vi "Ivium driver 1-02.vi"() -> ()   [LabVIEW 2020]
uses:
  <vilib>/Utility/file.llb/Write To Spreadsheet File (DBL).vi
  <vilib>/Utility/file.llb/Read From Spreadsheet File (DBL).vi
  Instance           3 25Saved   Ivium driver 1-02 .vi
  Instance           4 25Saved   Ivium driver 1-02 .vi
  Instance           2 25Saved   Ivium driver 1-02 .vi
  IVIUM_remdriver.lvlib
panel:
  out "Device serial number":string
  in  "Read device serial number":bool
  out "XY Graph":cluster{"Y":dbl[], "Y":dbl[]}[](graph)
  in  "Tab Control direct mode/method mode":enum32{"Direct Control", "Method control"}(tab)
  out "cell on":bool
  in  "Set Mux channel":i32
  in  "Tab Control Ac/external/bistat":enum32{"AC", "Extern", "BiStat"}(tab)
  in  "Amplitude":dbl caption="V" format="%_4f"
  in  "Frequency":dbl caption="Hz" format="%#_8f"
  out "Dig in 2":bool
  out "Dig in 1":bool
  in  "Dig out 1":bool
  in  "Read analog inputs":bool
  out "value /V":dbl[](array[numeric]) format="%_6g"
  in  "ch2":dbl caption="V" format="%_4g"
  in  "ch1":dbl caption="V" format="%_4p"
  in  "Read digital inputs":bool
  in  "Dig out 2":bool
  in  "Dig out 3":bool
  in  "Set Bi-Stat mode":enum16{"Standard", "Scanning"}(ring)
  in  "Get current":bool
  out "current 2":dbl caption="A" format="%_4g"
  in  "current range":T1(ring)=enum."1 mA"
  in  "offset potential":dbl caption="V" format="%_4g"
  in  "Get current":bool
  out "current":dbl caption="A" format="%_4g"
  in  "cell current":dbl caption="A" format="%_4p"
  in  "cell potential":dbl caption="V" format="%_3p"
  in  "Apply":enum16{"off", "on"}(ring)
  in  "Current range":T2(ring)=enum."10 mA"
  in  "Configuration":T3(ring)
  out "Device Status indicator":string
  in  "Get device status":bool
  out "cell-off button pressed":bool
  out "E_overload":bool
  out "Aninput1_overload":bool
  out "I_overload":bool
  in  "Get cell status":bool
  in  "Reset 2":bool
  out "potential":dbl caption="V" format="%_4g"
  in  "Get potential":bool
  in  "Set Filter":T4(ring)=enum."10 kHz"
  in  "Set Stability":T5(ring)=enum."Standard"
  in  "Reset 3":bool
  in  "Start/stop writing\ndata to spreadsheet file":bool
  in  "Start Chart":bool
  in  "Y Scale.Range:Minimum":dbl
  in  "Y Scale.Range:Maximum":dbl
  in  "stop":bool
  in  "Disconnect    Connect":bool
  # "I overload"
  # "Cell-off button pressed"
  # "E overload"
  # "Aninput1 overload"
  # "Ac signal"
  # "Analog input"
  # "Digital output"
  # "Analog output"
  # "ch1"
  # "ch2"
  # "ch3"
  # "ch4"
  # "ch5"
  # "Digital input"
  # "ch6"
  # "ch7"
  # "ch8"
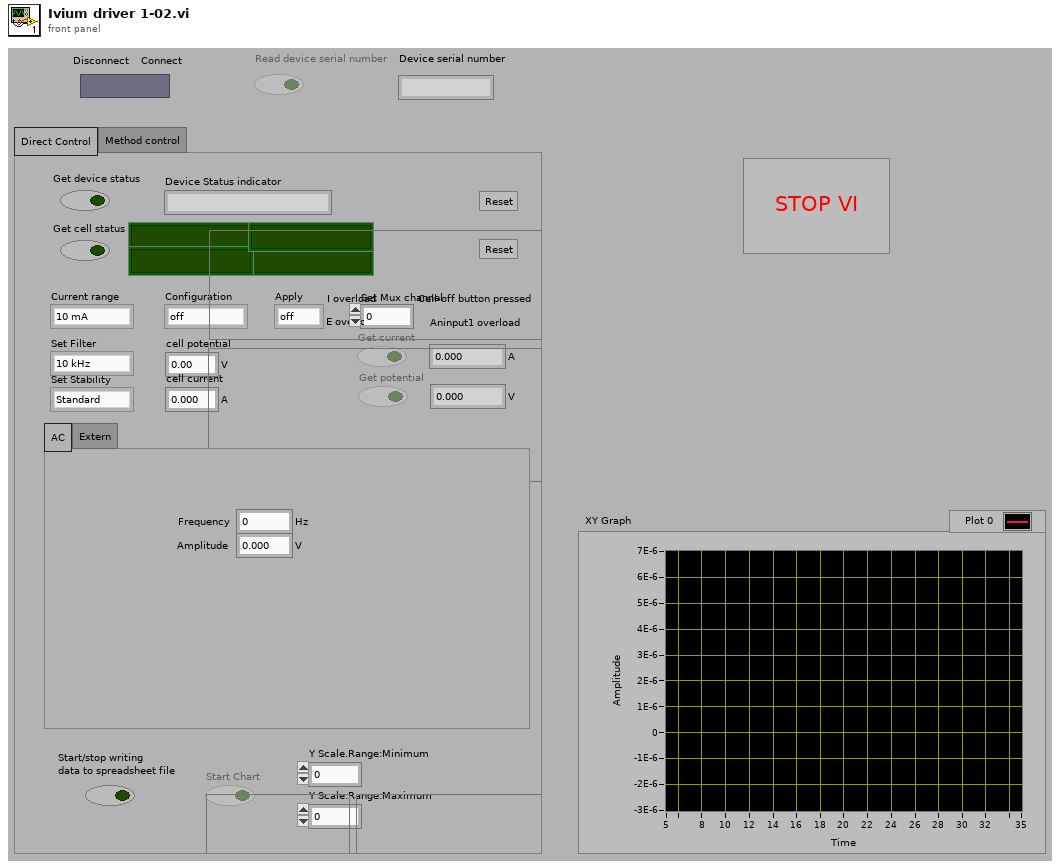
[diagram p1: front panel]
types:
  T1 = enum16{"10 mA", "1 mA", "100 uA", "10 uA", "1 uA", "100 nA", "10 nA", "1 nA", "100 pA", "10 pA", "1 pA"}
  T2 = enum16{"10 A", "1 A", "100 mA", "10 mA", "1 mA", "100 uA", "10 uA", "1 uA", "100 nA", "10 nA", "1 nA", "100 pA", "10 pA", "1 pA"}
  T3 = enum16{"off", "EStat4EL", "EStat2EL", "EStatDummy1", "EStatDummy2", "EStatDummy3", "EStatDummy4", "IStat4EL", "IStat2EL", "IStatDummy", "BiStat4EL", "BiStat2EL"}
  T4 = enum16{"1 MHz", "100 kHz", "10 kHz", "1 kHz", "10 Hz"}
  T5 = enum16{"High Speed", "Standard", "High Stability"}
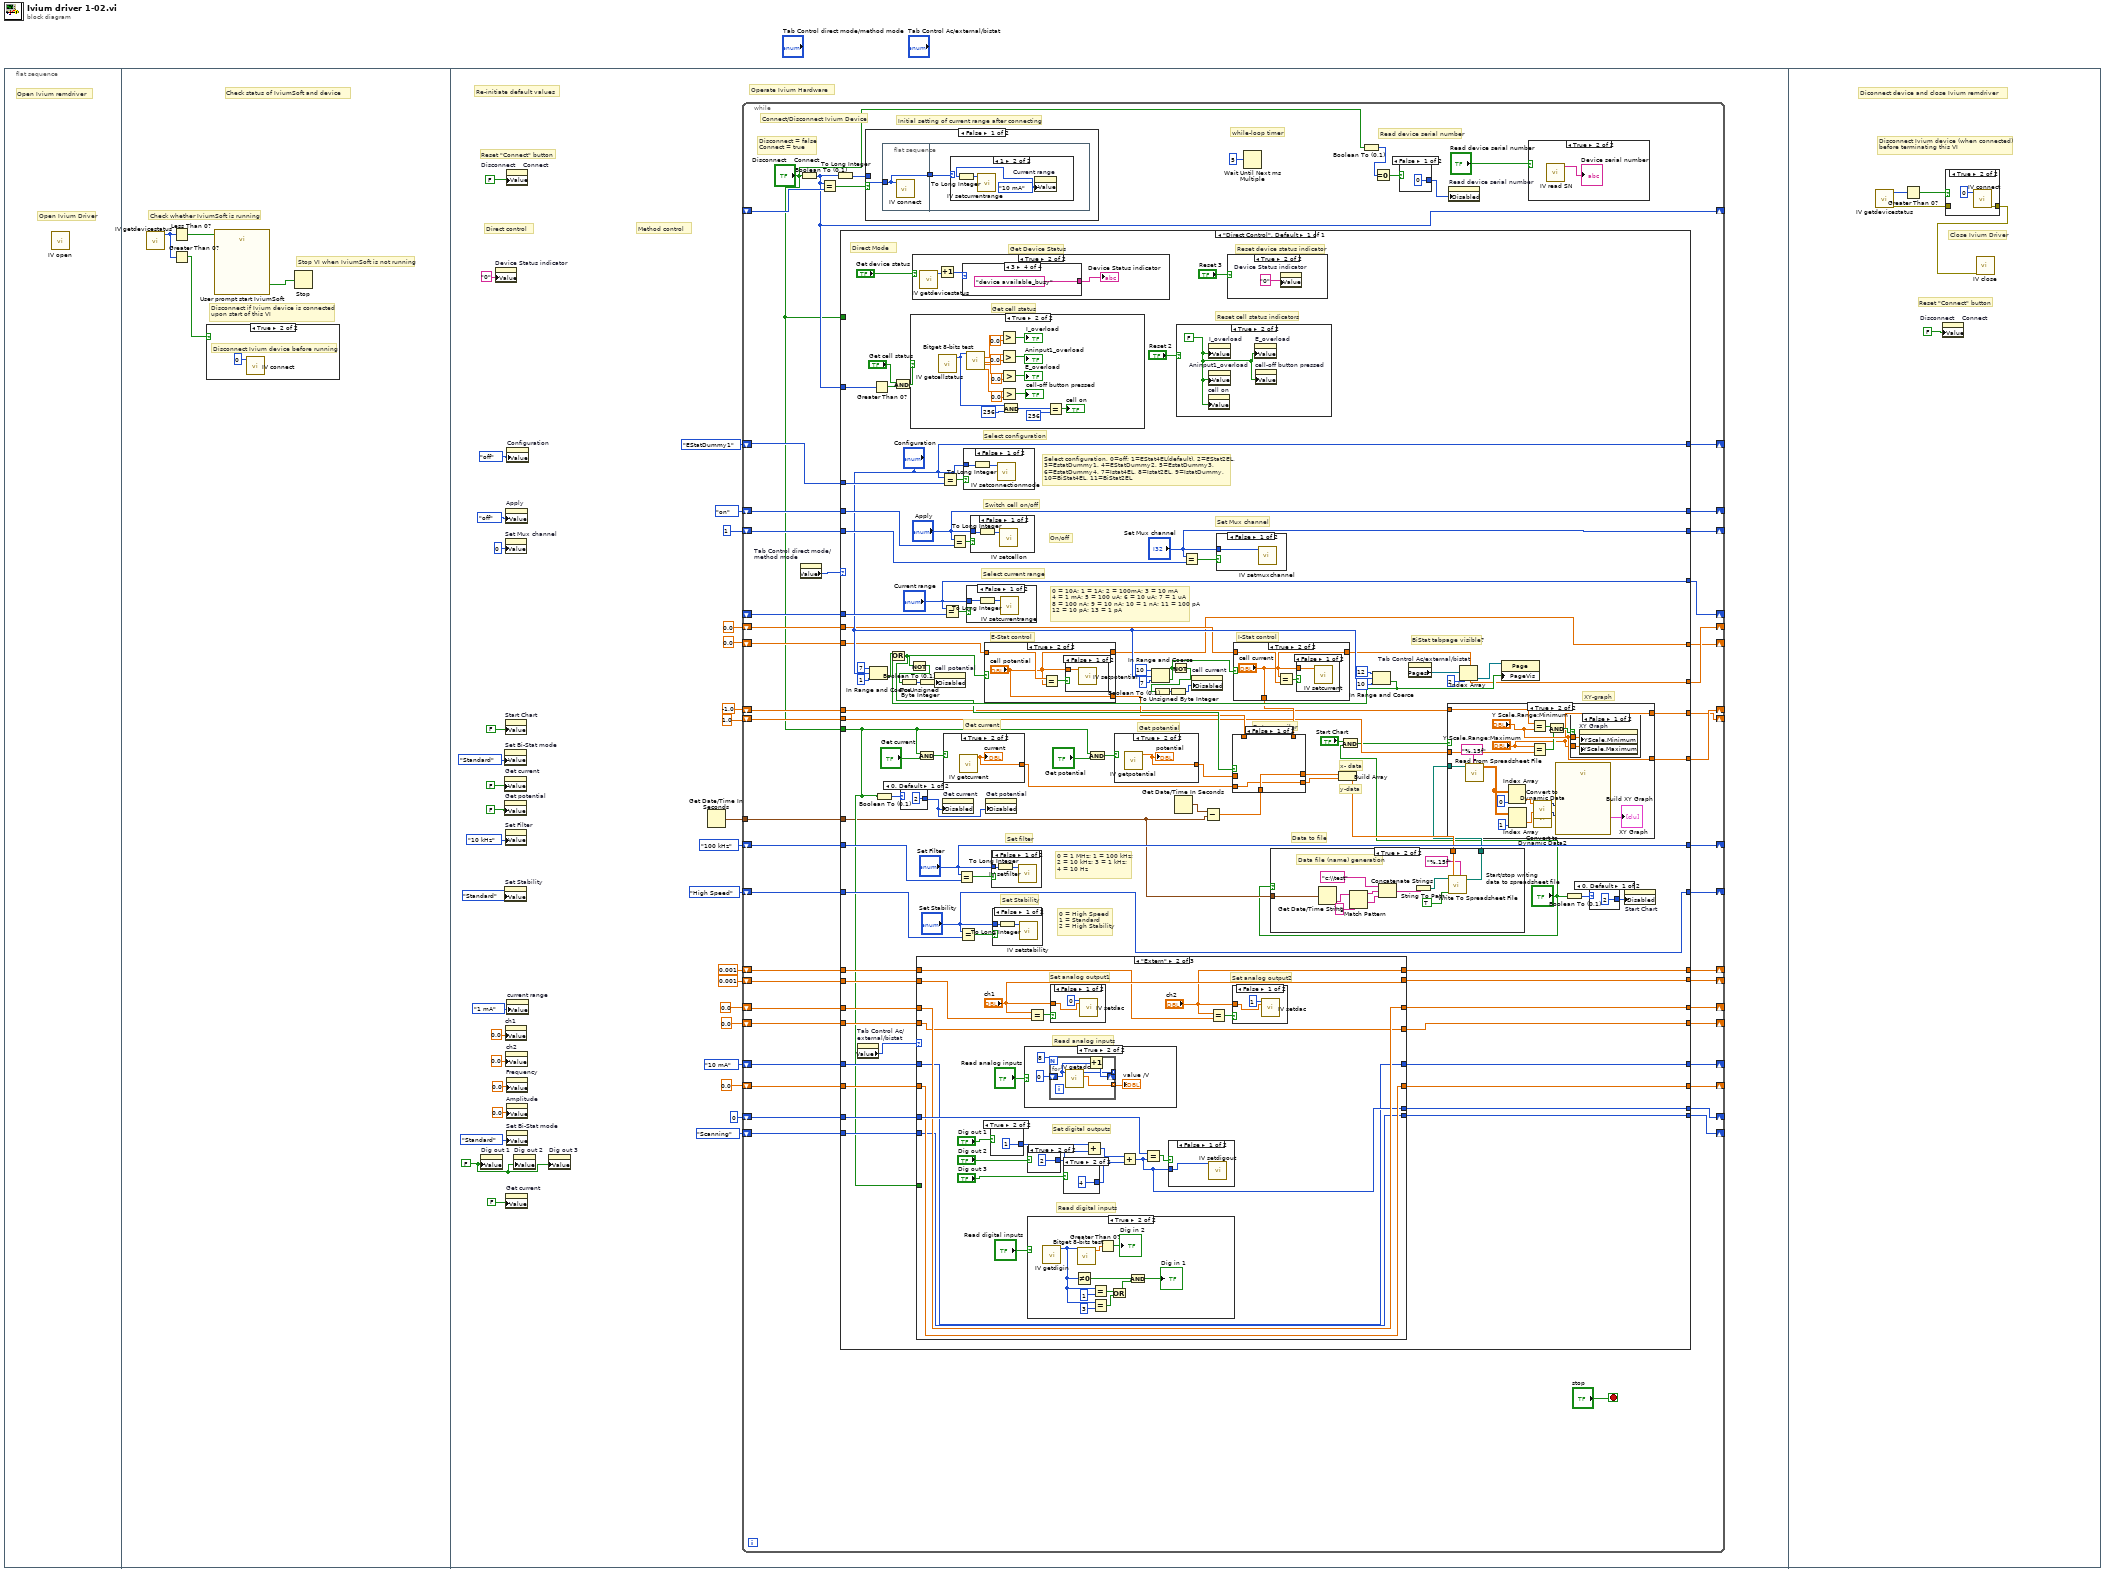
[diagram p0: block diagram]
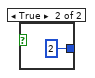
[diagram p4: hidden frame]
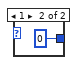
[diagram p5: hidden frame]
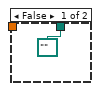
[diagram p6: hidden frame]
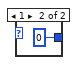
[diagram p10: hidden frame]
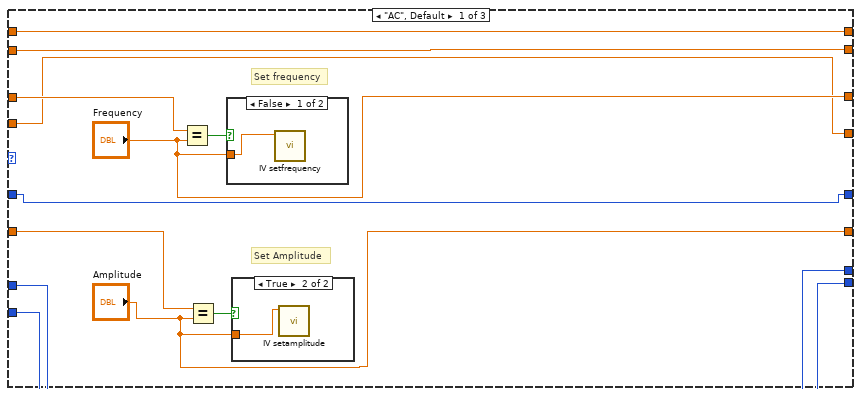
[diagram p12: hidden frame]
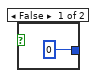
[diagram p16: hidden frame]
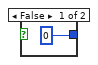
[diagram p17: hidden frame]
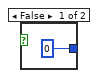
[diagram p18: hidden frame]
diagram:
  n1 = flat-sequence {
    frame #0 {
      # "Open Ivium remdriver"
      # "Open Ivium Driver"
      n2 = call "IV open.vi"() -> ()  [unwired: 10 in, 2 out]
    }
    frame #1 {
      # "Check status of IviumSoft and device"
      # "Stop VI when IviumSoft is not running"
      # "Disconnect if Ivium device is connected \nupon start of this VI"
      # "Check whether IviumSoft is running"
      n3 = call "IV getdevicestatus.vi"() -> ("return type"=w4:i32)  [unwired: 10 in, 1 out]
      n4 = Less Than 0?(x=w4) -> (x < 0?=w1:bool)
      n5 = Greater Than 0?(x=w4) -> (x > 0?=w3:bool)
      n6 = case shown="True" w3 {
        frame False {
        }
        frame True {
          # "Disconnect Ivium device before running"
          n7 = call "IV connect.vi"("devconnect"=0) -> ()  [unwired: 8 in, 3 out]
        }
      }
      n8 = call "User prompt start IviumSoft.vi"("Enable"=w1) -> ("OK"=w2:bool)  [unwired: 17 in, 1 out]
      n9 = Stop(stop? (T)=w2) -> ()
    }
    frame #2 {
      w12 = FALSE
      # "Method control"
      # "Direct control"
      # "Reset \"Connect\" button"
      # "Re-initiate default values"
      # "Operate Ivium Hardware"
      n10 = property on="Dig out 1" class="Bool (strict)"("Value"=w12) -> ()  [unwired: 2 in, 2 out]
      n11 = property on="Device Status indicator" class="Str"("Value"="0" ("Device Status indicator 2")) -> ()  [unwired: 2 in, 2 out]
      n12 = property on="Set Bi-Stat mode" class="Enum (strict)"("Value"=enum16{"Standard", "Scanning"}."Standard" ("Set Bi-Stat mode")) -> ()  [unwired: 2 in, 2 out]
      n13 = property on="Get current" class="Bool (strict)"("Value"=FALSE ("Get current")) -> ()  [unwired: 2 in, 2 out]
      n14 = property on="Get potential" class="Bool (strict)"("Value"=FALSE ("Get potential")) -> ()  [unwired: 2 in, 2 out]
      n15 = property on="Set Stability" class="Enum (strict)"("Value"=T5."Standard" ("Set Stability")) -> ()  [unwired: 2 in, 2 out]
      n16 = property on="Set Mux channel" class="DigNum (strict)"("Value"=0 ("Set Mux channel")) -> ()  [unwired: 2 in, 2 out]
      n17 = property on="Start Chart" class="Bool (strict)"("Value"=FALSE ("Start Chart")) -> ()  [unwired: 2 in, 2 out]
      n18 = property on="Set Filter" class="Enum (strict)"("Value"=T4."10 kHz" ("Set Filter")) -> ()  [unwired: 2 in, 2 out]
      n19 = property on="ch1" class="DigNum (strict)"("Value"=0.0 ("ch1")) -> ()  [unwired: 2 in, 2 out]
      n20 = property on="Apply" class="Enum (strict)"("Value"=enum16{"off", "on"}."off" ("Cell on/off")) -> ()  [unwired: 2 in, 2 out]
      n21 = property on="ch2" class="DigNum (strict)"("Value"=0.0 ("ch2")) -> ()  [unwired: 2 in, 2 out]
      n22 = property on="Get current" class="Bool (strict)"("Value"=FALSE ("Get current")) -> ()  [unwired: 2 in, 2 out]
      n23 = property on="Disconnect    Connect" class="Bool (strict)"("Value"=FALSE) -> ()  [unwired: 2 in, 2 out]
      n24 = property on="Frequency" class="DigNum (strict)"("Value"=0.0 ("Frequency")) -> ()  [unwired: 2 in, 2 out]
      n25 = property on="Amplitude" class="DigNum (strict)"("Value"=0.0 ("Amplitude")) -> ()  [unwired: 2 in, 2 out]
      n26 = property on="Set Bi-Stat mode" class="Enum (strict)"("Value"=enum16{"Standard", "Scanning"}."Standard" ("Set Bi-Stat mode")) -> ()  [unwired: 2 in, 2 out]
      n27 = property on="Configuration" class="Enum (strict)"("Value"=T3."off" ("Configuration")) -> ()  [unwired: 2 in, 2 out]
      n28 = property on="current range" class="Enum (strict)"("Value"=T1."1 mA" ("current range")) -> ()  [unwired: 2 in, 2 out]
      n29 = property on="Dig out 2" class="Bool (strict)"("Value"=w12) -> ()  [unwired: 2 in, 2 out]
      n30 = property on="Dig out 3" class="Bool (strict)"("Value"=w12) -> ()  [unwired: 2 in, 2 out]
      n31 = Get Date/Time In Seconds() -> (seconds since 1Jan1904=w9:timestamp)
      n32 = while {
        shift-right: [w61] -> _
        shift-left: _ -> [w91]
        shift-right: [w84] -> _
        shift-left: _ -> [w89]
        shift-right: [w87] -> _
        shift-left: T3."EStatDummy1" ("Configuration") -> [w88]
        shift-right: [w86] -> _
        shift-left: enum16{"off", "on"}."on" ("Apply") -> [w85]
        shift-right: [w82] -> _
        shift-left: T1."10 mA" ("current range") -> [w81]
        shift-right: [w79] -> _
        shift-left: T4."100 kHz" ("Set Filter") -> [w80]
        shift-right: [w77] -> _
        shift-left: T5."High Speed" ("Set Stability") -> [w78]
        shift-right: [w76] -> _
        shift-left: enum16{"Standard", "Scanning"}."Scanning" ("Set Bi-Stat mode") -> [w75]
        shift-right: [w73] -> _
        shift-left: 0.001 ("ch1") -> [w74]
        shift-right: [w72] -> _
        shift-left: 0.001 ("ch2") -> [w71]
        shift-right: [w70] -> _
        shift-left: 1 ("Set Mux channel") -> [w69]
        shift-right: [w60] -> _
        shift-left: 0 -> [w67]
        shift-right: [w65] -> _
        shift-left: 0.0 -> [w66]
        shift-right: [w63] -> _
        shift-left: 0.0 -> [w64]
        shift-right: [w58] -> _
        shift-left: 0.0 -> [w59]
        shift-right: [w56] -> _
        shift-left: 0.0 -> [w57]
        shift-right: [w54] -> _
        shift-left: 0.0 -> [w55]
        tunnel: w9 -> [w53]
        shift-right: [w50] -> _
        shift-left: -1.0 -> [w52]
        shift-right: [w49] -> _
        shift-left: 1.0 -> [w51]
        stop <- "stop" stop-if-true
        # "Read device serial number"
        # "while-loop timer"
        # "Initial setting of current range after connecting"
        # "Disconnect = false\nConnect = true"
        # "Connect/Disconnect Ivium Device"
        n33 = Boolean To (0,1)(Boolean="Disconnect    Connect") -> (0, 1=w61:i16)
        n34 = property on="Tab Control direct mode/\nmethod mode" class="TabCtl (strict)"() -> ("Value"=w48:enum32{"Direct Control", "Method control"})  [unwired: 2 in, 2 out]
        n35 = Equal?(x=w61, y=w91) -> (x = y?=w90:bool)
        n36 = To Long Integer(number=w61) -> (32bit integer=w62:i32)
        n37 = case shown="\"Direct Control\", Default" w48 {
          tunnel: w89 -> [w185]
          tunnel: w88 -> [w183]
          tunnel: ["Configuration"] -> w87
          tunnel: ["Apply"] -> w86
          tunnel: w85 -> [w180]
          tunnel: "Disconnect    Connect" -> [w123]
          tunnel: ["Current range"] -> w84
          tunnel: w61 -> [w169]
          tunnel: [w133] -> w82
          tunnel: w81 -> [w134]
          tunnel: w80 -> [w159]
          tunnel: ["Set Filter"] -> w79
          tunnel: w78 -> [w157]
          tunnel: ["Set Stability"] -> w77
          tunnel: [w131] -> w76
          tunnel: w75 -> [w132]
          tunnel: w74 -> [w155]
          tunnel: [w154] -> w73
          tunnel: [w153] -> w72
          tunnel: w71 -> [w152]
          tunnel: ["Set Mux channel"] -> w70
          tunnel: w69 -> [w150]
          tunnel: w67 -> [w145]
          tunnel: w66 -> [w144]
          tunnel: [w143] -> w65
          tunnel: w64 -> [w142]
          tunnel: [w141] -> w63
          tunnel: [w130] -> w60
          tunnel: w59 -> [w129]
          tunnel: [w128] -> w58
          tunnel: w57 -> [w114]
          tunnel: [w113] -> w56
          tunnel: w55 -> [w112]
          tunnel: [w111] -> w54
          tunnel: w53 -> [w106]
          tunnel: w52 -> [w105]
          tunnel: w51 -> [w104]
          tunnel: [w103] -> w50
          tunnel: [w102] -> w49
          tunnel: "Disconnect    Connect" -> [_]
          frame "Direct Control", Default {
            # "XY-graph"
            # "Data to file"
            # "Data compiler"
            # "y-data"
            # "x- data"
            # "BiStat tabpage visible?"
            # "Get potential"
            # "Get current"
            # "Set Mux channel"
            # "Reset device status indicator"
            # "0 = High Speed\n1 = Standard \n2 = High Stability"
            # "Set Stability"
            # "0 = 1 MHz; 1 = 100 kHz; \n2 = 10 kHz; 3 = 1 kHz; \n4 = 10 Hz"
            # "Set filter"
            # "On/off"
            # "I-Stat control"
            # "E-Stat control"
            # "Reset cell status indicators"
            # "Get cell status"
            # "Get Device Status"
            # "0 = 10A; 1 = 1A; 2 = 100mA; 3 = 10 mA\n4 = 1 mA; 5 = 100 uA; 6 = 10 uA; 7 = 1 uA\n8 = 100 nA; 9 = 10 nA; 10 = 1 nA; 11 = 100 pA\n12 = 10 pA; 13 = 1 pA"
            # "Select configuration"
            # "Direct Mode"
            # "Switch cell on/off"
            # "Select current range"
            # "Select configuration, 0=off; 1=EStat4EL(default), 2=EStat2EL, 3=EstatDummy1, 4=EStatDummy2, 5=EstatDummy3, 6=EstatDummy4, 7=Istat4EL, 8=Istat2EL, 9=IstatDummy, 10=BiStat4EL, 11=BiStat2EL"
            n38 = property on="Tab Control Ac/\nexternal/bistat" class="TabCtl (strict)"() -> ("Value"=w127:enum32{"AC", "Extern", "BiStat"})  [unwired: 2 in, 2 out]
            n39 = In Range and Coerce(upper limit=u16 7, x="Configuration", lower limit=u16 1) -> (In Range?=w162:bool)  [unwired: 1 out]
            n40 = Greater Than 0?(x=w169) -> (x > 0?=w170:bool)
            n41 = Boolean To (0,1)(Boolean=w123) -> (0, 1=w147:i16)
            n42 = And(x="Get cell status", y=w170) -> (x .and. y?=w172:bool)
            n43 = case shown="0, Default" w147 {
              tunnel: [u8 2 u8 0] -> w146
              frame 0, Default {
              }
              frame 1 {
              }
            }
            n44 = case shown="True" w172 {
              frame False {
              }
              frame True {
                n45 = call "IV getcellstatus.vi"() -> ("devcellstatus out"=w336:i32)  [unwired: 9 in, 2 out]
                n46 = call "Bitget 8-bits test.vi"("x"=w336) -> ("c"=w341:dbl, "e"=w339:dbl, "f"=w340:dbl, "h"=w337:dbl)  [unwired: 19 in, 4 out]
                n47 = Greater?(x=w341, y=0.0) -> (0:→"I_overload":bool)
                n48 = Greater?(x=w339, y=0.0) -> (0:→"Aninput1_overload":bool)
                n49 = Greater?(x=w340, y=0.0) -> (0:→"E_overload":bool)
                n50 = Greater?(x=w337, y=0.0) -> (0:→"cell-off button pressed":bool)
                n51 = And(x=w336, y=256) -> (x .and. y?=w334:i32)
                n52 = Equal?(x=w334, y=256) -> (x = y?=→"cell on":bool)
              }
            }
            n53 = case shown="True" "Get device status" {
              frame False {
                (unwired) 0
              }
              frame True {
                n54 = call "IV getdevicestatus.vi"() -> ("return type"=w351:i32)  [unwired: 10 in, 1 out]
                n55 = Increment(x=w351) -> (x+1=w350:i32)
                n56 = case shown="3" w350 {
                  tunnel: ["no IviumSoft" "device not connected" "device available_idle" "device available_busy"] -> w349
                  frame 0, Default {
                  }
                  frame 1 {
                  }
                  frame 2 {
                  }
                  frame 3 {
                  }
                }
                "Device Status indicator" <- w349
              }
            }
            n57 = case shown="\"Extern\"" w127 {
              tunnel: w155 -> [w240 w265 w306]
              tunnel: [w240 "ch1" w306] -> w154
              tunnel: [w241 "ch2" w307] -> w153
              tunnel: w152 -> [w241 w261 w307]
              tunnel: w145 -> [w231 w250 w303]
              tunnel: w144 -> [w238 w248 w305]
              tunnel: ["Frequency" w248 w305] -> w143
              tunnel: w142 -> [w235 w249 w304]
              tunnel: ["Amplitude" w249 w304] -> w141
              tunnel: w134 -> [w233 w245 w311]
              tunnel: [w233 w245 "current range"] -> w133
              tunnel: w132 -> [w232 w247 w309]
              tunnel: [w232 w247 "Set Bi-Stat mode"] -> w131
              tunnel: [w231 w246 w303] -> w130
              tunnel: w129 -> [w230 w244 w299]
              tunnel: [w230 w244 "offset potential"] -> w128
              tunnel: w123 -> [_ _ w295]
              frame "AC", Default {
                # "Set Amplitude"
                # "Set frequency"
                n58 = Equal?(x=w238, y="Frequency") -> (x = y?=w239:bool)
                n59 = Equal?(x=w235, y="Amplitude") -> (x = y?=w236:bool)
                n60 = case shown="False" w239 {
                  tunnel: "Frequency" -> [w243 _]
                  frame False {
                    n61 = call "IV setfrequency.vi"("value"=w243) -> ()  [unwired: 8 in, 3 out]
                  }
                  frame True {
                  }
                }
                n62 = case shown="True" w236 {
                  tunnel: "Amplitude" -> [_ w242]
                  frame False {
                  }
                  frame True {
                    n63 = call "IV setamplitude.vi"("value"=w242) -> ()  [unwired: 8 in, 3 out]
                  }
                }
              }
              frame "Extern" {
                # "Read digital inputs"
                # "Set digital outputs"
                # "Read analog inputs"
                # "Set analog output2"
                # "Set analog output1"
                n64 = case shown="True" "Dig out 1" {
                  tunnel: [0 1] -> w255
                  frame False {
                  }
                  frame True {
                  }
                }
                n65 = case shown="True" "Read analog inputs" {
                  frame False {
                  }
                  frame True {
                    n66 = for {
                      N: 8 -> [_]
                      shift-right: [w290] -> _
                      shift-left: 0 -> [w289]
                      tunnel: [w288] -> w284 mode=indexing
                      tunnel: [w287] -> _ mode=indexing
                      n67 = call "IV getadc.vi"("channr"=w289) -> ("value out"=w288:dbl, "channr out"=w287:i32)  [unwired: 7 in, 2 out]
                      n68 = Increment(x=w289) -> (x+1=w290:i32)
                    }
                    "value /V" <- w284
                  }
                }
                n69 = case shown="True" "Dig out 2" {
                  tunnel: [0 2] -> w254
                  frame False {
                  }
                  frame True {
                  }
                }
                n70 = case shown="True" "Read digital inputs" {
                  frame False {
                  }
                  frame True {
                    n71 = call "IV getdigin.vi"() -> ("value out"=w281:i32)  [unwired: 9 in, 2 out]
                    n72 = Not Equal To 0?(x=w281) -> (x != 0?=w276:bool)
                    n73 = call "Bitget 8-bits test.vi"("x"=w281) -> ("b"=w274:dbl)  [unwired: 19 in, 7 out]
                    n74 = Equal?(x=w281, y=1) -> (x = y?=w279:bool)
                    n75 = Equal?(x=w281, y=3) -> (x = y?=w278:bool)
                    n76 = Greater Than 0?(x=w274) -> (x > 0?=→"Dig in 2":bool)
                    n77 = Or(x=w279, y=w278) -> (x .or. y?=w277:bool)
                    n78 = And(x=w276, y=w277) -> (x .and. y?=→"Dig in 1":bool)
                  }
                }
                n79 = Equal?(x="ch1", y=w265) -> (x = y?=w266:bool)
                n80 = case shown="False" w266 {
                  tunnel: "ch1" -> [w293 _]
                  frame False {
                    n81 = call "IV setdac.vi"("value"=w293, "channr"=0) -> ()  [unwired: 6 in, 4 out]
                  }
                  frame True {
                  }
                }
                n82 = case shown="True" "Dig out 3" {
                  tunnel: [0 4] -> w252
                  frame False {
                  }
                  frame True {
                  }
                }
                n83 = Add(x=w255, y=w254) -> (x+y=w253:i32)
                n84 = Add(x=w253, y=w252) -> (x+y=w246:i32)
                n85 = Equal?(x=w250, y=w246) -> (x = y?=w251:bool)
                n86 = case shown="False" w251 {
                  tunnel: w246 -> [w267 _]
                  frame False {
                    n87 = call "IV setdigout.vi"("value"=w267) -> ()  [unwired: 8 in, 3 out]
                  }
                  frame True {
                  }
                }
                n88 = Equal?(x="ch2", y=w261) -> (x = y?=w263:bool)
                n89 = case shown="False" w263 {
                  tunnel: "ch2" -> [w291 _]
                  frame False {
                    n90 = call "IV setdac.vi"("value"=w291, "channr"=1) -> ()  [unwired: 6 in, 4 out]
                  }
                  frame True {
                  }
                }
              }
              frame "BiStat" {
                # "Bi-Stat mode:\n0 = standard\n1 = scanning"
                # "Bi-Stat current ranges:\n0 = 10 mA; 1 = 1 mA;\n2 = 100 uA; 3 = 10 uA;\n4 = 1 uA; 5 = 100 nA;\n6 = 10 nA; 7 = 1 nA;\n8 = 100 pA; 9 = 10 pA;\n10 = 1 pA"
                # "Bi-Stat control"
                n91 = Equal?(x=w299, y="offset potential") -> (x = y?=w300:bool)
                n92 = Equal?(x="current range", y=w311) -> (x = y?=w302:bool)
                n93 = Equal?(x="Set Bi-Stat mode", y=w309) -> (x = y?=w301:bool)
                n94 = case shown="True" w300 {
                  tunnel: "offset potential" -> [_ w313]
                  frame False {
                  }
                  frame True {
                    n95 = call "IV setpotential WE2.vi"("value"=w313) -> ()  [unwired: 8 in, 3 out]
                  }
                }
                n96 = case shown="False" w302 {
                  tunnel: "current range" -> [w316 _]
                  frame False {
                    n97 = To Long Integer(number=w316) -> (32bit integer=w317:i32)
                    n98 = call "IV setcurrentrange WE2.vi"("value"=w317) -> ()  [unwired: 8 in, 3 out]
                  }
                  frame True {
                  }
                }
                n99 = case shown="True" w301 {
                  tunnel: "Set Bi-Stat mode" -> [_ w314]
                  frame False {
                  }
                  frame True {
                    n100 = To Long Integer(number=w314) -> (32bit integer=w315:i32)
                    n101 = call "IV setbistatmode.vi"("value"=w315) -> ()  [unwired: 8 in, 3 out]
                  }
                }
                n102 = And(x=w295, y="Get current") -> (x .and. y?=w296:bool)
                n103 = case shown="True" w296 {
                  frame False {
                  }
                  frame True {
                    n104 = call "IV getcurrent WE2.vi"() -> ("value out"=→"current 2":dbl)  [unwired: 9 in, 2 out]
                  }
                }
              }
            }
            n105 = And(x=w123, y="Get current") -> (x .and. y?=w179:bool)
            n106 = Equal?(x="Configuration", y=w183) -> (x = y?=w184:bool)
            n107 = property on="Get current" class="Bool (strict)"("Disabled"=w146) -> ()  [unwired: 2 in, 2 out]
            n108 = Equal?(x="Current range", y=w185) -> (x = y?=w186:bool)
            n109 = case shown="True" w179 {
              tunnel: [0.0 ("value out") w363] -> w118
              frame False {
              }
              frame True {
                n110 = call "IV getcurrent.vi"() -> ("value out"=w363:dbl)  [unwired: 9 in, 2 out]
                "current" <- w363
              }
            }
            n111 = Equal?(x="Apply", y=w180) -> (x = y?=w182:bool)
            n112 = Equal?(x="Set Filter", y=w159) -> (x = y?=w122:bool)
            n113 = Equal?(x="Set Stability", y=w157) -> (x = y?=w158:bool)
            n114 = case shown="False" w184 {
              tunnel: "Configuration" -> [w366 _]
              frame False {
                n115 = To Long Integer(number=w366) -> (32bit integer=w367:i32)
                n116 = call "IV setconnectionmode.vi"("value"=w367) -> ()  [unwired: 8 in, 3 out]
              }
              frame True {
              }
            }
            n117 = case shown="False" w186 {
              tunnel: "Current range" -> [w368 _]
              frame False {
                n118 = To Long Integer(number=w368) -> (32bit integer=w369:i32)
                n119 = call "IV setcurrentrange.vi"("value"=w369) -> ()  [unwired: 8 in, 3 out]
              }
              frame True {
              }
            }
            n120 = case shown="False" w182 {
              tunnel: "Apply" -> [w364 _]
              frame False {
                n121 = To Long Integer(number=w364) -> (32bit integer=w365:i32)
                n122 = call "IV setcellon.vi"("cellon"=w365) -> ()  [unwired: 8 in, 3 out]
              }
              frame True {
              }
            }
            n123 = property on="Get potential" class="Bool (strict)"("Disabled"=w146) -> ()  [unwired: 2 in, 2 out]
            n124 = case shown="False" w122 {
              tunnel: "Set Filter" -> [w322 _]
              frame False {
                n125 = To Long Integer(number=w322) -> (32bit integer=w321:i32)
                n126 = call "IV setfilter.vi"("value"=w321) -> ()  [unwired: 8 in, 3 out]
              }
              frame True {
              }
            }
            n127 = case shown="False" w158 {
              tunnel: "Set Stability" -> [w320 _]
              frame False {
                n128 = To Long Integer(number=w320) -> (32bit integer=w319:i32)
                n129 = call "IV setstability.vi"("value"=w319) -> ()  [unwired: 8 in, 3 out]
              }
              frame True {
              }
            }
            n130 = And(x=w123, y="Get potential") -> (x .and. y?=w161:bool)
            n131 = case shown="True" w161 {
              tunnel: [0.0 ("value out") w324] -> w116
              frame False {
              }
              frame True {
                n132 = call "IV getpotential.vi"() -> ("value out"=w324:dbl)  [unwired: 9 in, 2 out]
                "potential" <- w324
              }
            }
            n133 = In Range and Coerce(upper limit=u16 10, x="Configuration", lower limit=u16 7) -> (In Range?=w165:bool)  [unwired: 1 out]
            n134 = Not(x=w165) -> (.not. x?=w137:bool)
            n135 = Boolean To (0,1)(Boolean=w137) -> (0, 1=w135:i16)
            n136 = To Unsigned Byte Integer(number=w135) -> (unsigned 8bit integer=w136:u8)
            n137 = Get Date/Time In Seconds() -> (seconds since 1Jan1904=w110:timestamp)
            n138 = case shown="True" "Reset 2" {
              frame False {
              }
              frame True {
                w331 = FALSE
                n139 = property on="cell on" class="Bool (strict)"("Value"=w331) -> ()  [unwired: 2 in, 2 out]
                n140 = property on="I_overload" class="Bool (strict)"("Value"=w331) -> ()  [unwired: 2 in, 2 out]
                n141 = property on="Aninput1_overload" class="Bool (strict)"("Value"=w331) -> ()  [unwired: 2 in, 2 out]
                n142 = property on="E_overload" class="Bool (strict)"("Value"=w331) -> ()  [unwired: 2 in, 2 out]
                n143 = property on="cell-off button pressed" class="Bool (strict)"("Value"=w331) -> ()  [unwired: 2 in, 2 out]
              }
            }
            n144 = Equal?(x="Set Mux channel", y=w150) -> (x = y?=w151:bool)
            n145 = property on="cell current" class="DigNum (strict)"("Disabled"=w136) -> ()  [unwired: 2 in, 2 out]
            n146 = Subtract(x=w110, y=w106) -> (x-y=w109:dbl)
            n147 = case shown="False" w151 {
              tunnel: "Set Mux channel" -> [w229 _]
              frame False {
                n148 = call "IV setmuxchannel.vi"("value"=w229) -> ()  [unwired: 8 in, 3 out]
              }
              frame True {
              }
            }
            n149 = case shown="True" "Reset 3" {
              frame False {
              }
              frame True {
                n150 = property on="Device Status indicator" class="Str"("Value"="0" ("Device Status indicator")) -> ()  [unwired: 2 in, 2 out]
              }
            }
            n151 = case shown="True" w165 {
              tunnel: [0.0 ("cell current") "cell current"] -> w117
              tunnel: w114 -> [_ w329]
              tunnel: [0.0 ("cell current") "cell current"] -> w113
              frame False {
              }
              frame True {
                n152 = Equal?(x="cell current", y=w329) -> (x = y?=w328:bool)
                n153 = case shown="False" w328 {
                  tunnel: "cell current" -> [w330 _]
                  frame False {
                    n154 = call "IV setcurrent.vi"("value"=w330) -> ()  [unwired: 8 in, 3 out]
                  }
                  frame True {
                  }
                }
              }
            }
            n155 = And(x="Start Chart", y="Start/stop writing\ndata to spreadsheet file") -> (x .and. y?=w96:bool)
            n156 = In Range and Coerce(upper limit=u16 12, x="Configuration", lower limit=u16 10) -> (In Range?=w121:bool)  [unwired: 1 out]
            n157 = Or(x=w162, y=w121) -> (x .or. y?=w120:bool)
            n158 = Not(x=w120) -> (.not. x?=w174:bool)
            n159 = Boolean To (0,1)(Boolean=w174) -> (0, 1=w139:i16)
            n160 = To Unsigned Byte Integer(number=w139) -> (unsigned 8bit integer=w140:u8)
            n161 = property on="cell potential" class="DigNum (strict)"("Disabled"=w140) -> ()  [unwired: 2 in, 2 out]
            n162 = case shown="True" w120 {
              tunnel: [0.0 ("cell potential") "cell potential"] -> w119
              tunnel: w112 -> [_ w359]
              tunnel: [0.0 ("cell potential") "cell potential"] -> w111
              frame False {
              }
              frame True {
                n163 = Equal?(x=w359, y="cell potential") -> (x = y?=w360:bool)
                n164 = case shown="False" w360 {
                  tunnel: "cell potential" -> [w361 _]
                  frame False {
                    n165 = call "IV setpotential.vi"("value"=w361) -> ()  [unwired: 8 in, 3 out]
                  }
                  frame True {
                  }
                }
              }
            }
            n166 = case shown="False" w120 {
              tunnel: w119 -> [_ _]
              tunnel: [w202 w205] -> w100
              tunnel: w118 -> [w202 w205]
              tunnel: w117 -> [_ _]
              tunnel: w116 -> [_ _]
              tunnel: [w203 w204] -> w115
              tunnel: w109 -> [w203 w204]
              frame False {
              }
              frame True {
              }
            }
            n167 = Build Array(w115, w100) -> (w108:dbl[])
            n168 = case shown="True" "Start/stop writing\ndata to spreadsheet file" {
              tunnel: w108 -> [_ w201]
              tunnel: [path "" ("new file path (Not A Path if cancelled)") w199] -> w101
              tunnel: w106 -> [_ w191]
              frame False {
              }
              frame True {
                # "Data file (name) generation"
                n169 = Get Date/Time String(seconds (now)=w191) -> (time string=w195:string)  [unwired: 2 in, 1 out]
                n170 = Match Pattern(string=w195, regular expression=":") -> (before substring=w193:string, after substring=w192:string)  [unwired: 1 in, 2 out]
                n171 = Concatenate Strings("c:\\test", w193, w192) -> (w197:string)
                n172 = String To Path(string=w197) -> (path=w196:path)
                n173 = call-poly <vilib>:"Write To Spreadsheet File.vi"("format (%.3f)"="%.15f", "append to file? (new file:F)"=TRUE, "1D data"=w201, "file path (dialog if empty)"=w196) -> ("new file path (Not A Path if cancelled)"=w199:path)  [unwired: 4 in]
              }
            }
            n174 = property on="Tab Control Ac/external/bistat" class="TabCtl (strict)"() -> ("Pages"=w126:refnum<vi>[])  [unwired: 2 in, 2 out]
            n175 = case shown="True" w96 {
              tunnel: w105 -> [w206 w217]
              tunnel: w104 -> [w207 w211]
              tunnel: [w206 "Y Scale.Range:Minimum"] -> w103
              tunnel: [w207 "Y Scale.Range:Maximum"] -> w102
              tunnel: w101 -> [_ w209]
              frame False {
              }
              frame True {
                n176 = call-poly <vilib>:"Read From Spreadsheet File.vi"("format (%.3f)"="%.15f", "file path (dialog if empty)"=w209) -> ("all rows"=w210:dbl[][])  [unwired: 5 in, 4 out]
                n177 = Index Array(array=w210, index (col)=0 ("disabled index (col)")) -> (element=w222:dbl[])  [unwired: 1 in]
                n178 = Index Array(array=w210, index (col)=1 ("disabled index (col)")) -> (element=w219:dbl[])  [unwired: 1 in]
                n179 = Equal?(x=w217, y="Y Scale.Range:Minimum") -> (x = y?=w215:bool)
                n180 = Equal?(x="Y Scale.Range:Maximum", y=w211) -> (x = y?=w213:bool)
                n181 = call "Convert to Dynamic Data"("Array"=w222) -> ("Dynamic Data Type"=w221:dynamicdata)  [unwired: 3 in]
                n182 = call "Convert to Dynamic Data2"("Array"=w219) -> ("Dynamic Data Type"=w218:dynamicdata)  [unwired: 3 in]
                n183 = And(x=w215, y=w213) -> (x .and. y?=w214:bool)
                n184 = call "Build XY Graph"("Y Input"=w218, "X Input"=w221) -> ("XY Graph"=→"XY Graph":cluster{"Y":dbl[], "Y":dbl[]}[])  [unwired: 8 in, 1 out]
                n185 = case shown="False" w214 {
                  tunnel: "Y Scale.Range:Minimum" -> [w226 _]
                  tunnel: "Y Scale.Range:Maximum" -> [w225 _]
                  frame False {
                    n186 = property on="XY Graph" class="XYGraph (strict)"("YScale.Minimum"=w226, "YScale.Maximum"=w225) -> ()  [unwired: 2 in, 2 out]
                  }
                  frame True {
                  }
                }
              }
            }
            n187 = Index Array(array=w126, index=2) -> (element=w124:refnum<vi>)
            n188 = property class="Page"(reference=w124, "PageVis"=w121) -> ()  [unwired: 1 in, 2 out]
            n189 = Boolean To (0,1)(Boolean="Start/stop writing\ndata to spreadsheet file") -> (0, 1=w99:i16)
            n190 = case shown="0, Default" w99 {
              tunnel: [u8 2 u8 0] -> w98
              frame 0, Default {
              }
              frame 1 {
              }
            }
            n191 = property on="Start Chart" class="Bool (strict)"("Disabled"=w98) -> ()  [unwired: 2 in, 2 out]
          }
        }
        n192 = case shown="False" w90 {
          tunnel: w62 -> [w371 _]
          frame False {
            n193 = flat-sequence {
              tunnel: w371 -> [w372]
              tunnel: [w372] -> w370
              tunnel: w370 -> [w373]
              frame #0 {
                n194 = call "IV connect.vi"("devconnect"=w372) -> ()  [unwired: 8 in, 3 out]
              }
              frame #1 {
                n195 = case shown="1" w373 {
                  frame 0, Default {
                  }
                  frame 1 {
                    w374 = T2."10 mA" ("Current range selector")
                    n196 = To Long Integer(number=w374) -> (32bit integer=w375:i32)
                    n197 = call "IV setcurrentrange.vi"("value"=w375) -> ()  [unwired: 8 in, 3 out]
                    n198 = property on="Current range" class="Enum (strict)"("Value"=w374) -> ()  [unwired: 2 in, 2 out]
                  }
                }
              }
            }
          }
          frame True {
          }
        }
        n199 = Wait Until Next ms Multiple(millisecond multiple=u32 5 ("milliseconds to wait")) -> ()  [unwired: 1 out]
        n200 = Boolean To (0,1)(Boolean="Disconnect    Connect") -> (0, 1=w47:i16)
        n201 = Equal To 0?(x=w47) -> (x = 0?=w46:bool)
        n202 = case shown="False" w46 {
          tunnel: [u8 0 u8 2] -> w44
          frame False {
          }
          frame True {
          }
        }
        n203 = property on="Read device serial number" class="Bool"("Disabled"=w44) -> ()  [unwired: 2 in, 2 out]
        n204 = case shown="True" "Read device serial number" {
          frame False {
          }
          frame True {
            n205 = call "IV read SN.vi"() -> ("sntext out"=→"Device serial number":string)  [unwired: 9 in, 2 out]
          }
        }
      }
    }
    frame #3 {
      # "Diconnect device and close Ivium remdriver"
      # "Reset \"Connect\" button"
      # "Disconnect Ivium device (when connected)\nbefore terminating this VI"
      # "Close Ivium Driver"
      n206 = call "IV getdevicestatus.vi"() -> ("error out"=w377:errorcluster, "return type"=w379:i32)  [unwired: 10 in]
      n207 = Greater Than 0?(x=w379) -> (x > 0?=w378:bool)
      n208 = property on="Disconnect    Connect" class="Bool (strict)"("Value"=FALSE) -> ()  [unwired: 2 in, 2 out]
      n209 = case shown="True" w378 {
        tunnel: [w381 w382] -> w380
        tunnel: w377 -> [w381 _]
        frame False {
        }
        frame True {
          n210 = call "IV connect.vi"("devconnect"=0) -> ("error out"=w382:errorcluster)  [unwired: 8 in, 2 out]
        }
      }
      n211 = call "IV close.vi"("error in (no error)"=w380) -> ()  [unwired: 9 in, 2 out]
    }
  }
